vi "create voltage output command.vi"(9 "new output (V)":fxp<+/-,20,5>, 11 "channel":i32) -> (3 "command message":variant)   [LabVIEW 2018]
types:
  T1 = cluster{"channel":i32, "output Value":fxp<+/-,20,5>}
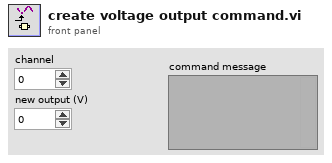
[diagram p1: front panel]
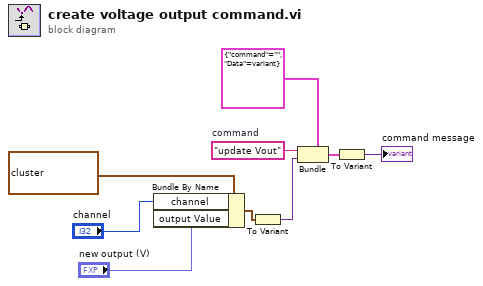
[diagram p0: block diagram]
diagram:
  w7 = "update Vout"  # command
  n1 = Bundle By Name(cluster=T1 {"channel"=0, "output Value"=0.0}, "channel"="channel", "output Value"="new output (V)") -> (w9:T1)
  n2 = To Variant(anything=w9) -> (Variant=w6:variant)
  n3 = Bundle(cluster=cluster{"command":string, "Data":variant} {"command"="", "Data"=variant}, "command"=w7, "Data"=w6) -> (w5:cluster{"command":string, "Data":variant})
  n4 = To Variant(anything=w5) -> (Variant=→"command message":variant)
